vi "SWLDA_Matrix_Constructor.vi"(0 "SWLDA_Matrix":path, 1 "ERP_Target":path, 2 "ERP_Nontarget":path, 5 "Weight_SWLDA":path, 7 "in":path, 12 "penter":dbl=0.4, 13 "premove":dbl=0.5, 14 "DIscard Channel Info":i32[](array[numeric])) -> ()   [LabVIEW 2014]
uses:
  <vilib>/Utility/file.llb/Read From Spreadsheet File (DBL).vi
  <vilib>/Utility/file.llb/Write To Spreadsheet File (DBL).vi
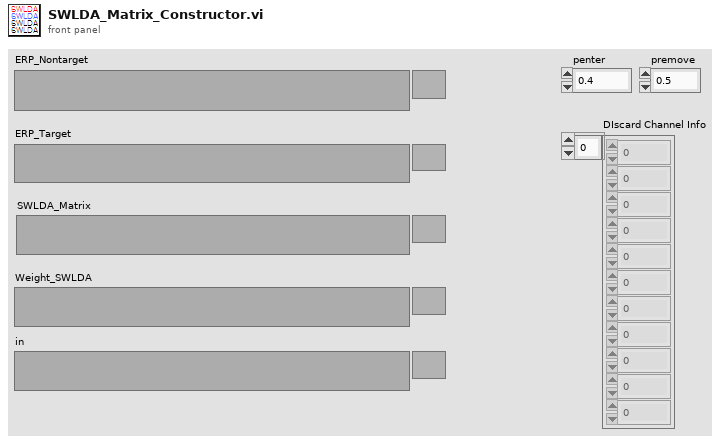
[diagram p1: front panel]
types:
  T1 = typedef "NI_Matrix.lvlib/RealMatrix.ctl" = dbl[][]
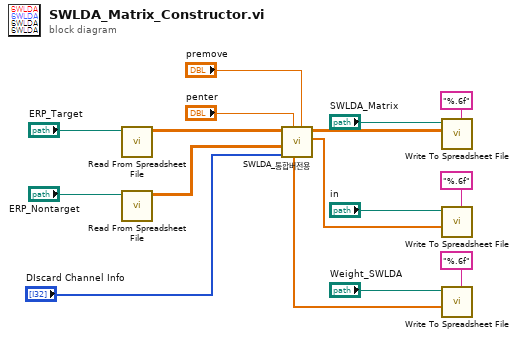
[diagram p0: block diagram]
diagram:
  n1 = call-poly <vilib>:"Read From Spreadsheet File.vi"("file path (dialog if empty)"="ERP_Target") -> ("all rows"=w16:dbl[][])  [unwired: 6 in, 4 out]
  n2 = call-poly <vilib>:"Read From Spreadsheet File.vi"("file path (dialog if empty)"="ERP_Nontarget") -> ("all rows"=w2:dbl[][])  [unwired: 6 in, 4 out]
  n3 = call "SWLDA_통합버전용.vi"("premove"="premove", "penter"="penter", "DIscard Channel Info"="DIscard Channel Info", "ERP_Nontarget"=w2, "ERP_Target"=w16) -> ("in"=w3:dbl[], "LDA_matrix"=w15:T1, "WEIGHT"=w12:dbl[])  [unwired: 4 in]
  n4 = call-poly <vilib>:"Write To Spreadsheet File.vi"("format (%.3f)"="%.6f", "2D data"=w15, "file path (dialog if empty)"="SWLDA_Matrix") -> ()  [unwired: 5 in, 1 out]
  n5 = call-poly <vilib>:"Write To Spreadsheet File.vi"("format (%.3f)"="%.6f", "1D data"=w3, "file path (dialog if empty)"="in") -> ()  [unwired: 5 in, 1 out]
  n6 = call-poly <vilib>:"Write To Spreadsheet File.vi"("format (%.3f)"="%.6f", "1D data"=w12, "file path (dialog if empty)"="Weight_SWLDA") -> ()  [unwired: 5 in, 1 out]
